vi "sub_SDR_mimo_AddPilots.vi"(9 "Port":enum16{"Port 1", "Port 2"}(ring), 10 "Array in":cdb[](array[numeric]), 11 "Symbols/Pilots":i32) -> (2 "Array Out":cdb[](array[numeric]))   [LabVIEW 2012]
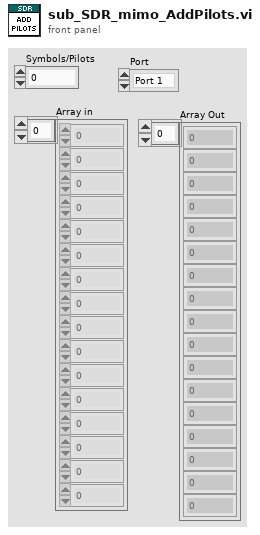
[diagram p1: front panel]
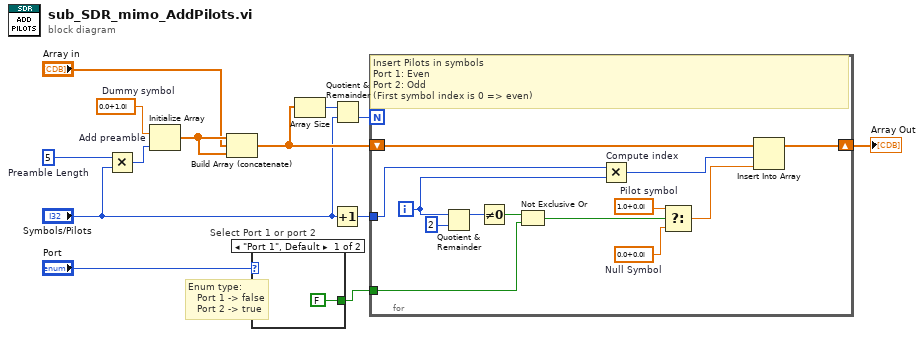
[diagram p0: block diagram]
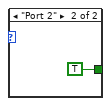
[diagram p2: hidden frame]
diagram:
  w1 = 5  # Preamble Length
  w7 = cdb 0.0+1.0i  # Dummy symbol
  # "Enum type:\n   Port 1 -> false\n   Port 2 -> true"
  n1 = Multiply(x=w1, y="Symbols/Pilots") -> (x*y=w3:i32)
  n2 = Initialize Array "Add preamble"(w7, w3) -> (w13:cdb[])
  n3 = Build Array (concatenate) "Build Array"(w13, "Array in", w13) -> (w9:cdb[])
  n4 = case "Select Port 1 or port 2" shown="\"Port 1\", Default" "Port" {
    tunnel: [FALSE ("x") TRUE ("x")] -> w4
    frame "Port 1", Default {
    }
    frame "Port 2" {
    }
  }
  n5 = Array Size(array=w9) -> (size(s)=w11:i32)
  n6 = Increment(x="Symbols/Pilots") -> (x+1=w6:i32)
  n7 = Quotient & Remainder(x=w11, y="Symbols/Pilots") -> (floor(x/y)=w10:i32)  [unwired: 1 out]
  n8 = for {
    N: w10 -> [_]
    tunnel: w6 -> [w27]
    shift-right: [w25] -> w12
    shift-left: w9 -> [w28]
    tunnel: w4 -> [w22]
    i -> [w24]
    w17 = cdb 0.0+0.0i  # Null Symbol
    w18 = cdb 1.0+0.0i  # Pilot symbol
    # "Insert Pilots in symbols\nPort 1: Even\nPort 2: Odd\n(First symbol index is 0 => even)"
    n9 = Quotient & Remainder(x=w24, y=2) -> (x-y*floor(x/y)=w21:i32)  [unwired: 1 out]
    n10 = Not Equal To 0?(x=w21) -> (x != 0?=w19:bool)
    n11 = Not Exclusive Or(1:w22, 2:w19) -> (0:w20:bool)
    n12 = Multiply "Compute index"(x=w27, y=w24) -> (x*y=w26:i32)
    n13 = Select(t=w18, s=w20, f=w17) -> (s? t:f=w16:cdb)
    n14 = Insert Into Array "Insert Into Array"(array=w28, index=w26, new element=w16) -> (w25:cdb[])
  }
  "Array Out" <- w12
